vi "LogWrite.vi"(8 "Error In":errorcluster, 10 "Setup":T1={"DUT"={"Count"=1, "Wirings"=[], "Names"=[]}, "Log"={"Start"={"Trigger Type"=enum."Immediate", "Timer (sec)"=0.0, "Digital IO Line"=0, "Digital IO Edge"=enum."Rising"}, "Rollover"={"Trigger Type"=enum."None", "Timer (sec)"=0.0, "File Size (MB)"=0, "Digital IO Line"=0, "Digital IO Edge"=enum."Rising"}, "Stop"={"Trigger Type"=enum."None", "Timer (sec)"=0.0, "File Size (MB)"=0, "Digital IO Line"=0, "Digital IO Edge"=enum."Rising"}}, "Trigger"={"Input"={"Type"=enum."None", "Timeout (ms)"=0, "Delay (ms)"=0, "Digital IO Line (1-14)"=0, "Digital IO Mode"=enum."Falling"}, "Output"={"Type"=enum."None", "Delay (ms)"=0, "Digital IO Line (1-14)"=0, "Digital IO Mode"=enum."Falling", "Digital IO Pulse Width (sec)"=0.0}}, "Sources"=[], "Measures"=[]} {"Measures"."Count" min=1 step=1; "Trigger"."Output"."Digital IO Line (1-14)" min=1 max=14 step=1}, 11 "Log Data":refnum<queue>) -> (0 "Error Out":errorcluster, 2 "Rearm?":bool, 3 "Rollover?":bool)   [LabVIEW 2012]
uses:
  Setup.ctl
  DUTConfiguration.ctl
  driver/Public/Controls/SMUSense.ctl
  LogConfiguration.ctl
  LogStartConfiguration.ctl
  LogStartTriggerType.ctl
  LogDigitalIOTriggerEdge.ctl
  LogRolloverConfiguration.ctl
  LogRolloverTriggerType.ctl
  LogStopConfiguration.ctl
  LogStopTriggerType.ctl
  TriggerConfiguration.ctl
  TriggerInputConfiguration.ctl
  TriggerInputType.ctl
  driver/Public/Controls/TriggerMode.ctl
  TriggerOutputConfiguration.ctl
  TriggerOutputType.ctl
  SourceConfiguration.ctl
  SourceFunction.ctl
  MeasureConfiguration.ctl
  HardwareLogData.ctl
  HardwareDisplayData.ctl
  LogFileGlobalAction.ctl
  driver/Keithley-2602.lvlib
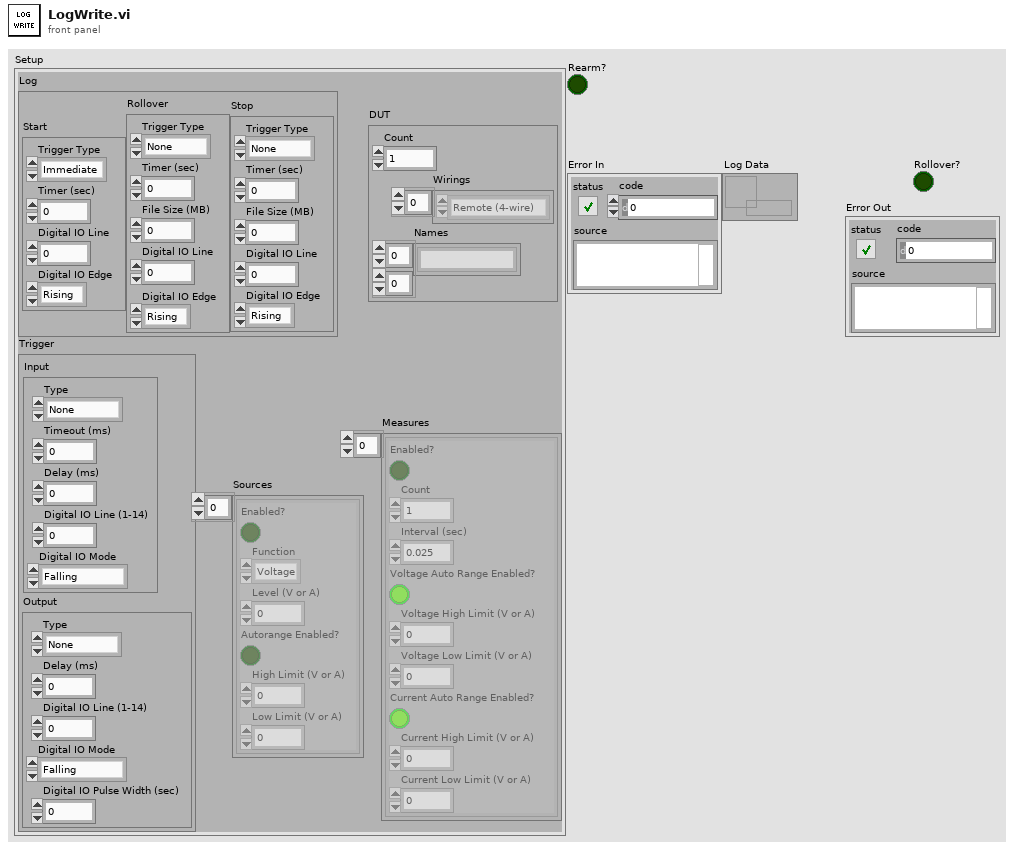
[diagram p1: front panel]
types:
  T1 = typedef "Setup.ctl" = cluster{"DUT":T2, "Log":T4, "Trigger":T12, "Sources":T18[], "Measures":T20[]}
  T2 = typedef "DUTConfiguration.ctl" = cluster{"Count":u32, "Wirings":T3[], "Names":string[][]}
  T3 = typedef "Keithley-2602.lvlib/SMUSense.ctl" = enum16{"Local (2-wire)", "Remote (4-wire)", "Calibration"}
  T4 = typedef "LogConfiguration.ctl" = cluster{"Start":T5, "Rollover":T8, "Stop":T10}
  T5 = typedef "LogStartConfiguration.ctl" = cluster{"Trigger Type":T6, "Timer (sec)":dbl, "Digital IO Line":u8, "Digital IO Edge":T7}
  T6 = typedef "LogStartTriggerType.ctl" = enum16{"Immediate", "User", "Timer", "Digital IO"}
  T7 = typedef "LogDigitalIOTriggerEdge.ctl" = enum16{"Rising", "Falling"}
  T8 = typedef "LogRolloverConfiguration.ctl" = cluster{"Trigger Type":T9, "Timer (sec)":dbl, "File Size (MB)":u32, "Digital IO Line":u8, "Digital IO Edge":T7}
  T9 = typedef "LogRolloverTriggerType.ctl" = enum16{"None", "Timer", "File Size", "Digital IO"}
  T10 = typedef "LogStopConfiguration.ctl" = cluster{"Trigger Type":T11, "Timer (sec)":dbl, "File Size (MB)":u32, "Digital IO Line":u8, "Digital IO Edge":T7}
  T11 = typedef "LogStopTriggerType.ctl" = enum16{"None", "User", "Timer", "File Size", "Digital IO"}
  T12 = typedef "TriggerConfiguration.ctl" = cluster{"Input":T13, "Output":T16}
  T13 = typedef "TriggerInputConfiguration.ctl" = cluster{"Type":T14, "Timeout (ms)":u32, "Delay (ms)":u32, "Digital IO Line (1-14)":u8, "Digital IO Mode":T15}
  T14 = typedef "TriggerInputType.ctl" = enum16{"None", "Digital IO", "Bus"}
  T15 = typedef "Keithley-2602.lvlib/TriggerMode.ctl" = enum16{"Falling", "Rising", "Either", "Synchronous"}
  T16 = typedef "TriggerOutputConfiguration.ctl" = cluster{"Type":T17, "Delay (ms)":u32, "Digital IO Line (1-14)":u8, "Digital IO Mode":T15, "Digital IO Pulse Width (sec)":dbl}
  T17 = typedef "TriggerOutputType.ctl" = enum16{"None", "Digital IO", "Bus"}
  T18 = typedef "SourceConfiguration.ctl" = cluster{"Enabled?":bool, "Function":T19, "Level (V or A)":dbl, "Autorange Enabled?":bool, "High Limit (V or A)":dbl, "Low Limit (V or A)":dbl}
  T19 = typedef "SourceFunction.ctl" = enum16{"Voltage", "Current"}
  T20 = typedef "MeasureConfiguration.ctl" = cluster{"Enabled?":bool, "Count":u8, "Interval (sec)":dbl, "Voltage Auto Range Enabled?":bool, "Voltage High Limit (V or A)":dbl, "Voltage Low Limit (V or A)":dbl, "Current Auto Range Enabled?":bool, "Current High Limit (V or A)":dbl, "Current Low Limit (V or A)":dbl}
  T21 = typedef "LogFileGlobalAction.ctl" = enum16{"Open", "Write", "Size", "Close"}
  T22 = typedef "HardwareLogData.ctl" = cluster{"Timestamp":timestamp, "Data":T23}
  T23 = typedef "HardwareDisplayData.ctl" = cluster{"DUT Names":string[][], "SMU":dbl[][], "Port":bool[]}
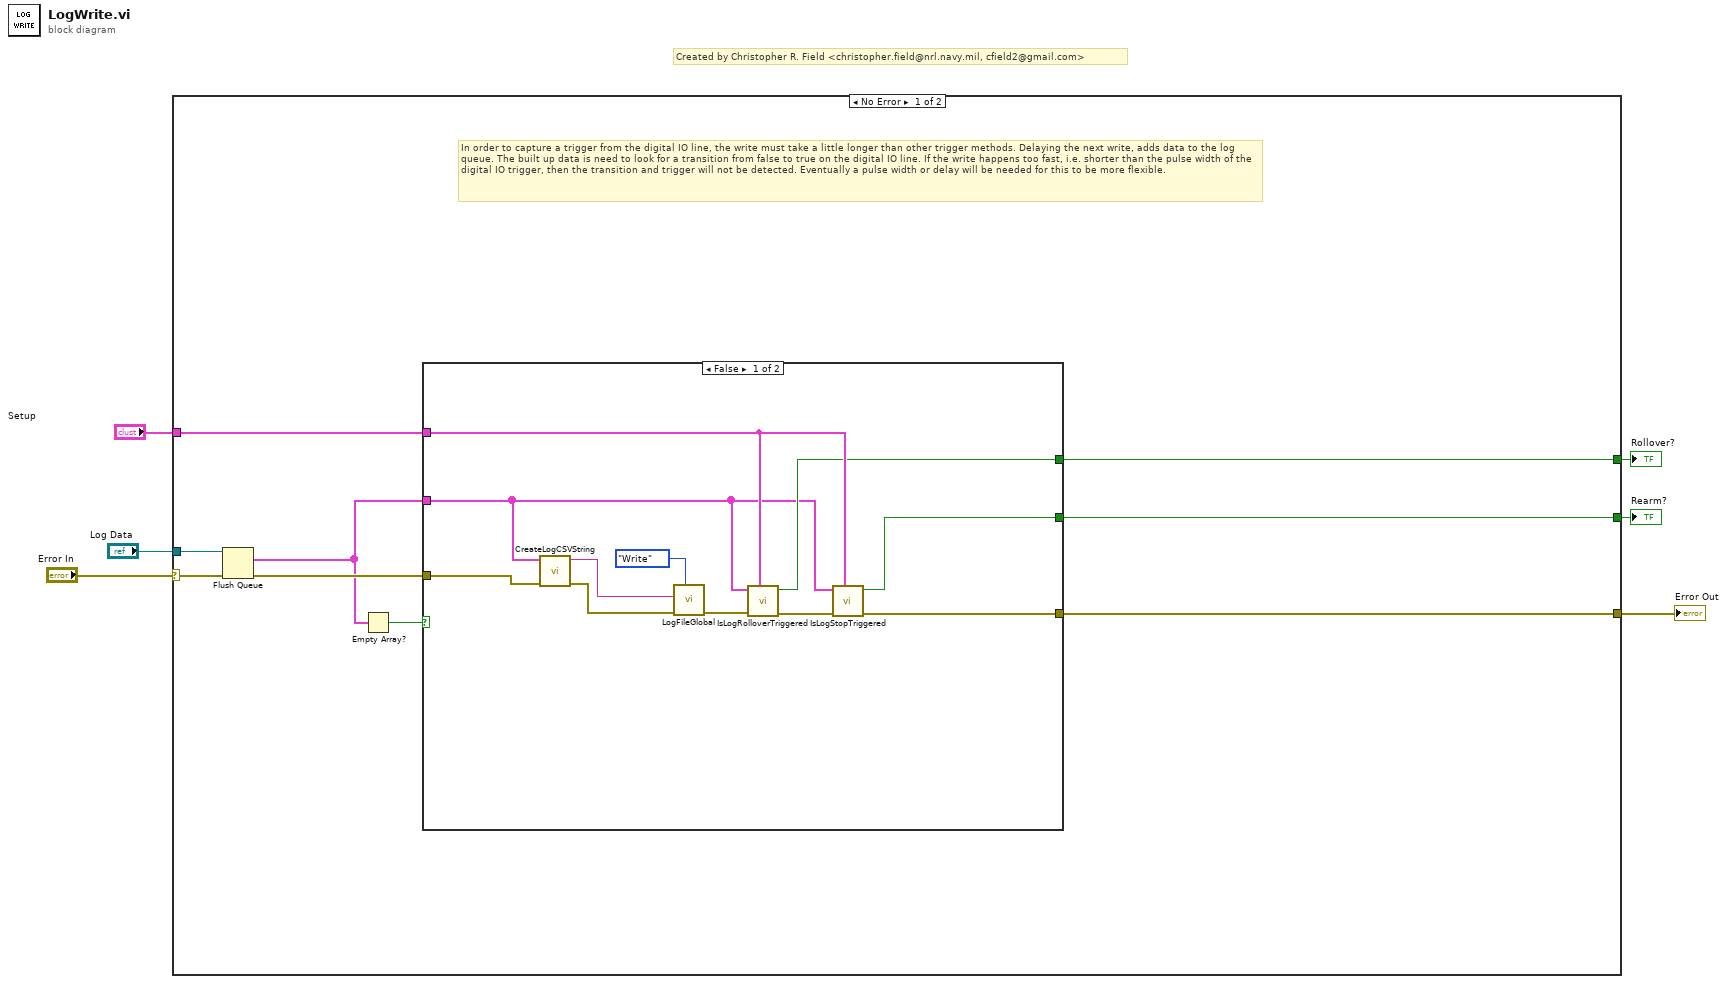
[diagram p0: block diagram]
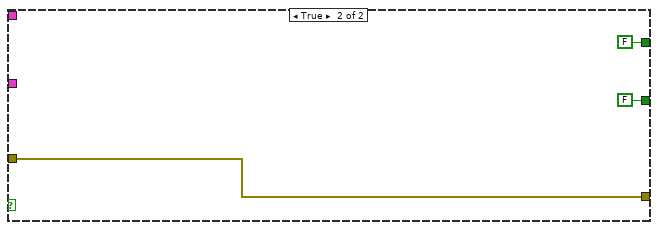
[diagram p2: hidden frame]
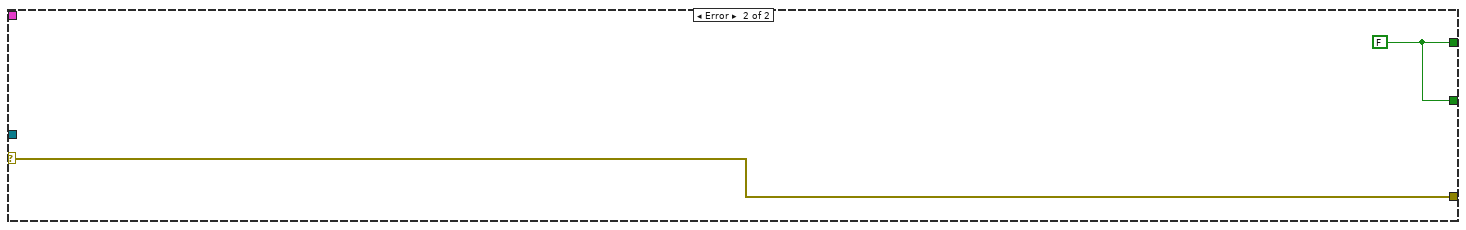
[diagram p3: hidden frame]
diagram:
  # "Created by Christopher R. Field <christopher.field@nrl.navy.mil, cfield2@gmail.com>"
  n1 = case shown="No Error" "Error In" {
    selector: "Error In" -> [w10 w31]
    tunnel: "Setup" -> [w14 _]
    tunnel: [w13 w31] -> w4
    tunnel: [w15 w30] -> w3
    tunnel: "Log Data" -> [w11 _]
    tunnel: [w12 w30] -> w1
    frame No Error {
      # "In order to capture a trigger from the digital IO line, the write must take a little longer than other trigger methods. Delaying the next write, adds data to the log queue. The built up data is need to look for a transition from false to true on the digital IO line. If the write happens too fast, i.e. shorter than the pulse width of the digital IO trigger, then the transition and trigger will not be detected. Eventually a pulse width or delay will be needed for this to be more flexible."
      n2 = Flush Queue(queue=w11, error in (no error)=w10) -> (remaining elements=w8:T22[], error out=w9:errorcluster)  [unwired: 1 out]
      n3 = Empty Array?(array=w8) -> (empty?=w7:bool)
      n4 = case shown="False" w7 {
        tunnel: [w18 FALSE ("Triggered?")] -> w15
        tunnel: w14 -> [w25 _]
        tunnel: [w24 w27] -> w13
        tunnel: [w17 FALSE ("Triggered?")] -> w12
        tunnel: w9 -> [w23 w27]
        tunnel: w8 -> [w16 _]
        frame False {
          n5 = call "CreateLogCSVString.vi"("Error In"=w23, "Log Data"=w16) -> ("Error Out"=w20:errorcluster, "CSV String"=w21:string)  [unwired: 8 in]
          n6 = call "LogFileGlobal.vi"("Action"=LogFileGlobalAction."Write", "Error In"=w20, "CSV String"=w21) -> ("Error Out"=w19:errorcluster)  [unwired: 7 in, 1 out]
          n7 = call "IsLogRolloverTriggered.vi"("Application Configuration"=w25, "Error In"=w19, "Log Data"=w16) -> ("Error Out"=w26:errorcluster, "Triggered?"=w18:bool)  [unwired: 7 in]
          n8 = call "IsLogStopTriggered.vi"("Application Configuration"=w25, "Error In"=w26, "Log Data"=w16) -> ("Error Out"=w24:errorcluster, "Triggered?"=w17:bool)  [unwired: 7 in]
        }
        frame True {
        }
      }
    }
    frame Error {
      w30 = FALSE ("Rollover?")
    }
  }
  "Error Out" <- w4
  "Rollover?" <- w3
  "Rearm?" <- w1
